vi "ClsSendInitCmds.vi"(8 "error in (no error)":errorcluster, 10 "InitCommandArray":string[](array[string]), 11 "Connection Out in":u32) -> (0 "error out":errorcluster, 2 "Array of Command Responses":string[](array[string]), 3 "Connection Out out":u32)   [LabVIEW 2015]
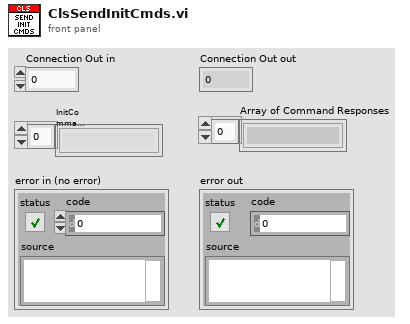
[diagram p1: front panel]
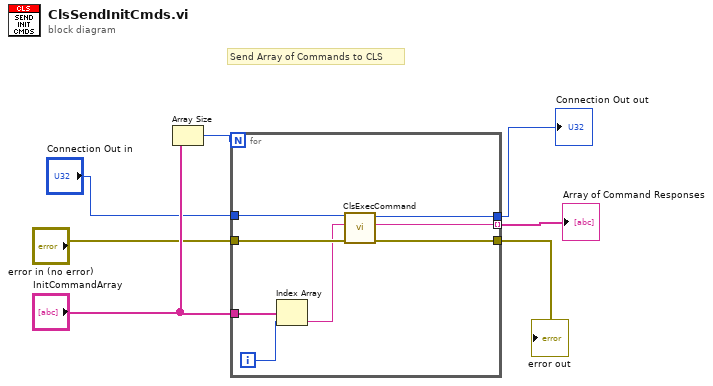
[diagram p0: block diagram]
diagram:
  # "Send Array of Commands to CLS"
  n1 = Array Size(array="InitCommandArray") -> (size(s)=w6:i32)
  n2 = for {
    N: w6 -> [_]
    tunnel: "error in (no error)" -> [w15]
    tunnel: [w14] -> w3
    tunnel: [w13] -> w4
    tunnel: "Connection Out in" -> [w12]
    tunnel: "InitCommandArray" -> [w10]
    tunnel: [w8] -> w1 mode=indexing
    i -> [w11]
    n3 = Index Array(array=w10, index=w11) -> (element=w9:string)
    n4 = call "ClsExecCommand.vi"("error in (no error)"=w15, "Command In"=w9, "Connection In"=w12) -> ("error out"=w14:errorcluster, "Command Response"=w8:string, "Connection Out"=w13:u32)  [unwired: 6 in]
  }
  "Connection Out out" <- w4
  "error out" <- w3
  "Array of Command Responses" <- w1
